vi "Measurement Logic.vi"(8 "error in":errorcluster, 9 "measurement configuration":T2 {"Baudrate" format="%x"; "FD Baudrate" format="%x"}, 10 "measure call context in":refnum<class "Measure Call Context.lvclass">, 11 "Stop OOB Server UE":refnum<user-event>) -> (0 "error out":errorcluster, 1 "measurement results":T1, 2 "measure call context out":refnum<class "Measure Call Context.lvclass">)   [LabVIEW 2025, in "CAN-LIN Raw Bus Capture.lvclass"]
doc: "Contains the core logic for executing the measurement."
uses:
  CAN-LIN Raw Bus Capture.lvclass
  <vilib>/Plug-In SDKs/Measurements/Measure Call Context/Measure Call Context.lvclass
  Measurement Configuration.ctl
  CAN-LIN Raw Bus Capture UI/Toggle.ctl
  Measurement Results.ctl
  <vilib>/xnet/xnet.llb/XNET Read (Frame LIN).vi
  CAN-LIN Raw Bus Capture.lvclass/CAN-LIN Raw Bus Capture.ctl
  <vilib>/xnet/xnet.llb/XNET Read (Frame CAN).vi
  OOB Data Transfer/OOB Data Transfer.lvlib
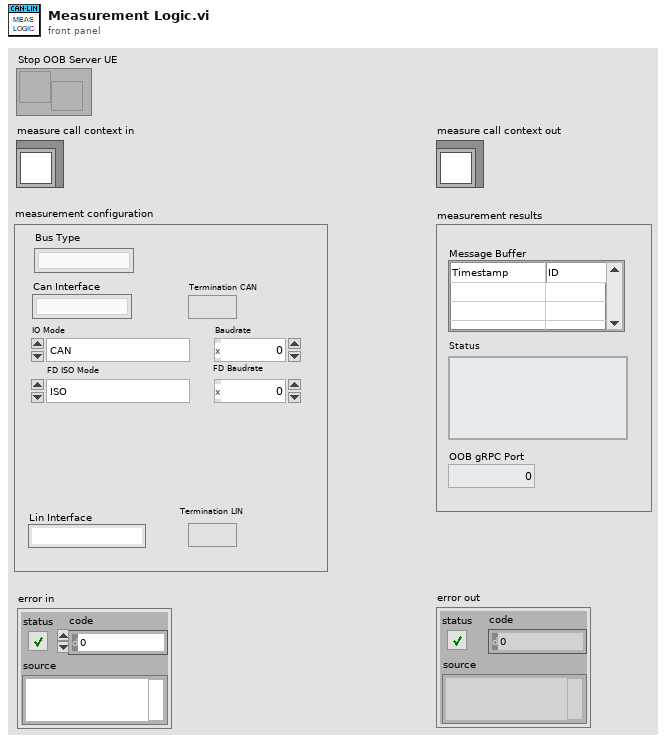
[diagram p1: front panel]
types:
  T1 = typedef "CAN-LIN Raw Bus Capture.lvclass/Measurement Results.ctl" = cluster{"Message Buffer":string[][], "Status":string, "OOB gRPC Port":i32}
  T2 = typedef "CAN-LIN Raw Bus Capture.lvclass/Measurement Configuration.ctl" = cluster{"Termination CAN":T3, "FD Baudrate":u32, "Baudrate":u32, "FD ISO Mode":enum32{"ISO", "Legacy ISO", "Non-ISO"}, "IO Mode":enum32{"CAN", "CAN FD", "CAN FD + BRS"}, "Termination LIN":T3, "Can Interface":string, "Lin Interface":string, "Bus Type":string}
  T3 = typedef "Toggle.ctl" = bool
  T4 = typedef "OOB Data Transfer.lvlib/OOB to Logic Data.ctl" = cluster{"PauseResume":bool, "Export":string}
  T5 = typedef "XNET Frame CAN.ctl" = cluster{"timestamp":timestamp, "payload":u8[], "identifier":u32, "type":T6, "extended?":bool, "echo?":bool}
  T6 = typedef "XNET Frame Type CAN.ctl" = u8
  T7 = typedef "XNET Frame LIN.ctl" = cluster{"timestamp":timestamp, "payload":u8[], "identifier":u32, "type":T8, "event ID":u8, "event slot?":bool, "echo?":bool}
  T8 = typedef "XNET Frame Type LIN.ctl" = u8
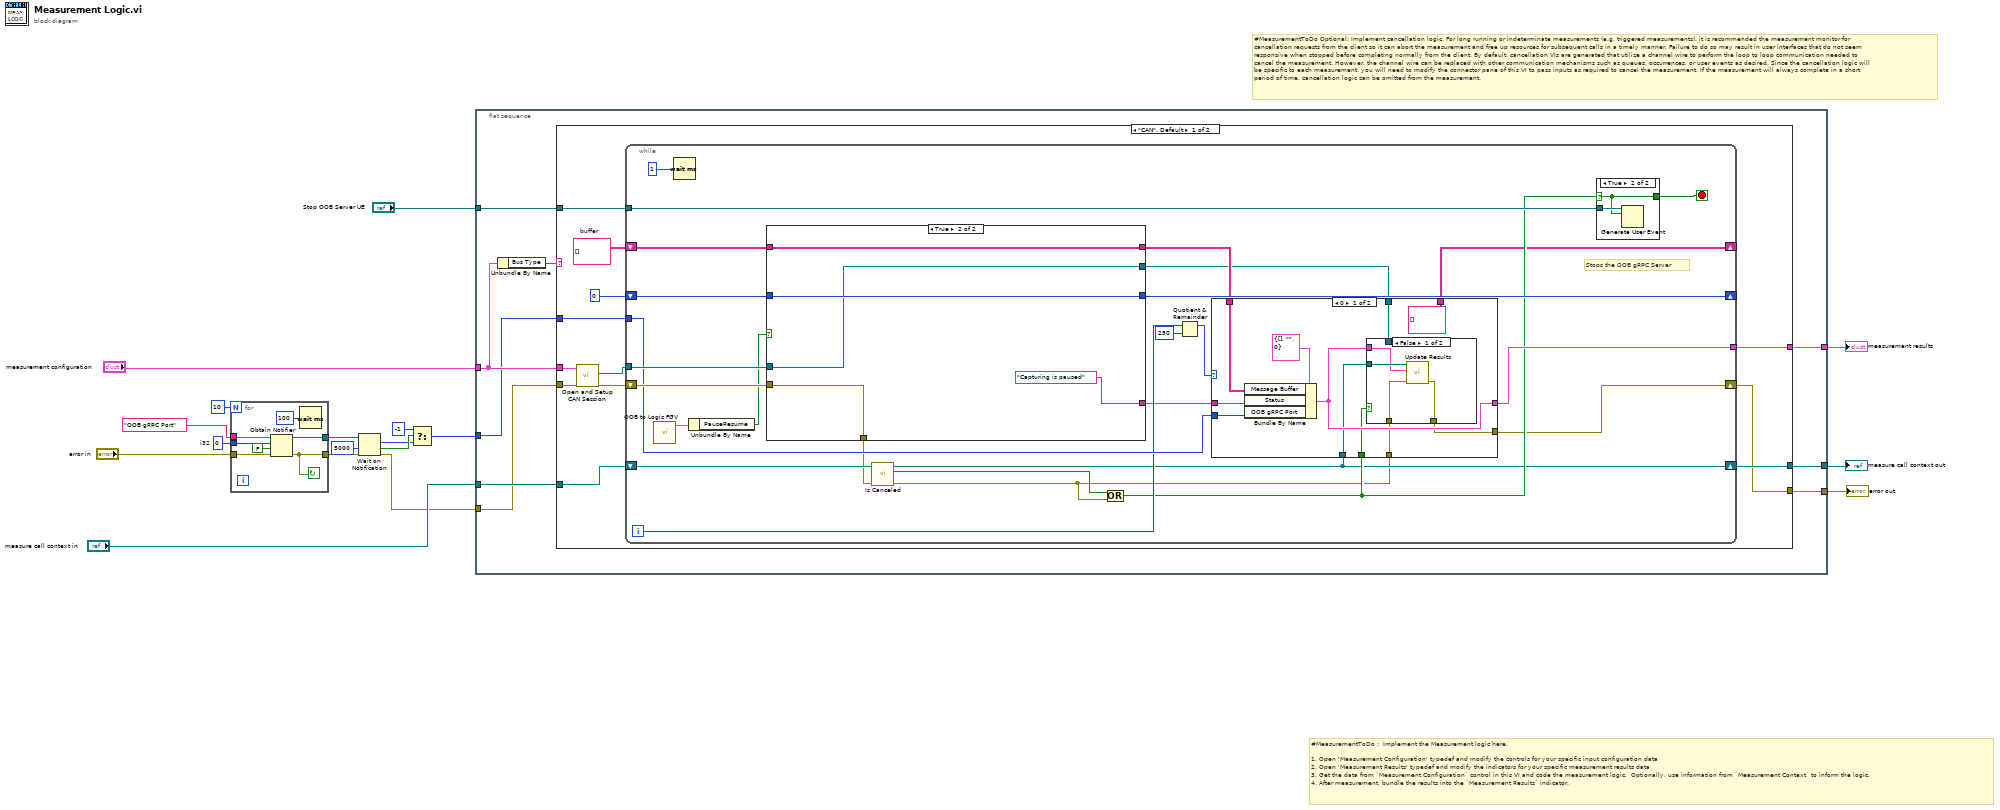
[diagram p0: block diagram]
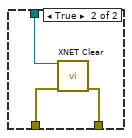
[diagram p2: hidden frame]
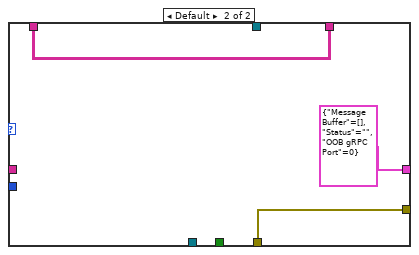
[diagram p3: hidden frame]
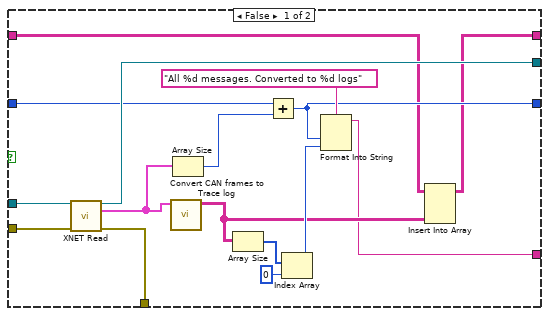
[diagram p4: hidden frame]
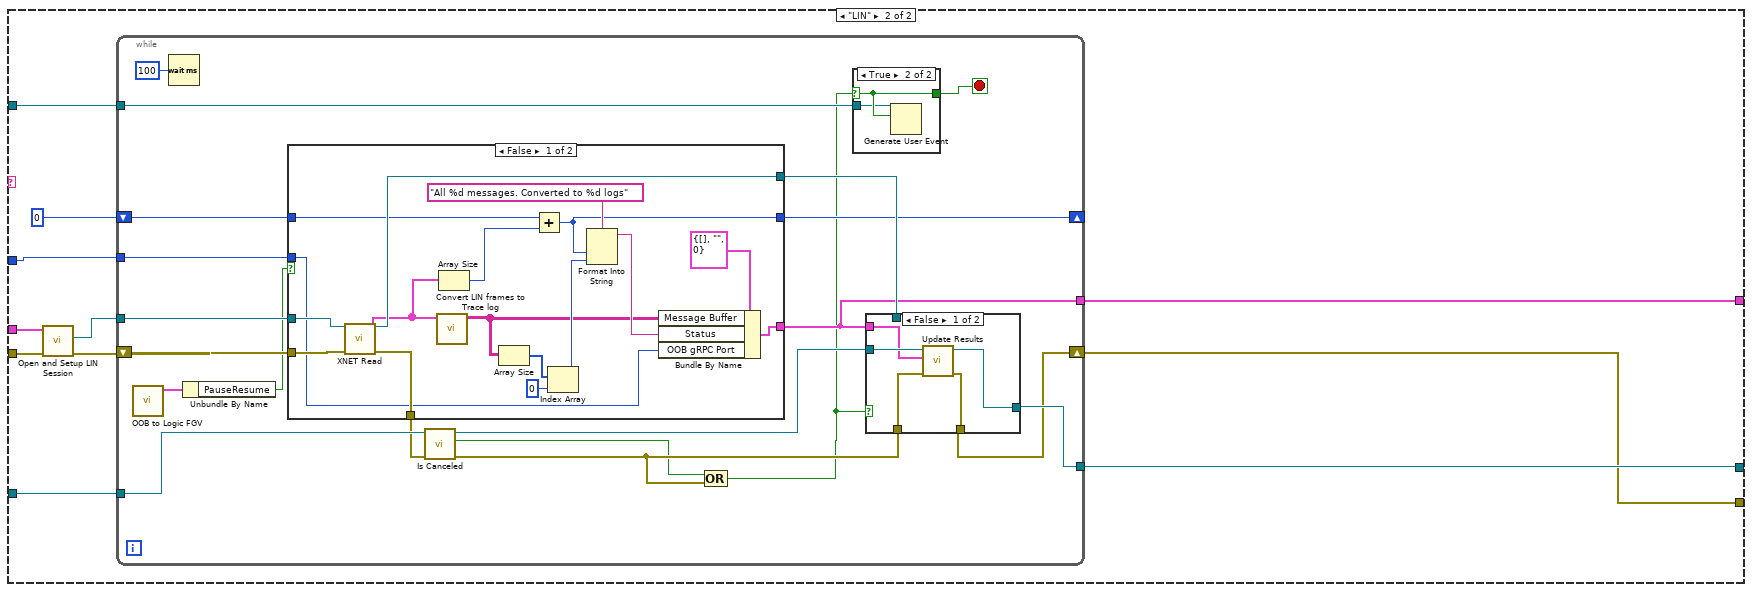
[diagram p6: hidden frame]
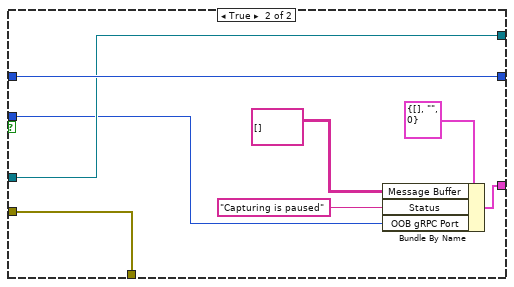
[diagram p8: hidden frame]
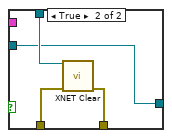
[diagram p9: hidden frame]
diagram:
  w8 = 0  # i32
  # "#MeasurementToDo Optional: Implement cancellation logic. For long running or indeterminate measurements (e.g. triggered measurements), it is recommended the measurement monitor for cancellation requests from the client so it can abort the measurement and free up resources for subsequent calls in a timely manner. Failure to do so may result in user interfaces that do not seem responsive when stopped before completing normally from the client. By default, cancellation VIs are generated that utilize a channel wire to perform the loop to loop communication needed to cancel the measurement. However, the channel wire can be replaced with other communication mechanisms such as queues, occurrences, or user events as desired. Since the cancellation logic will be specific to each measurement, you will need to modify the connector pane of this VI to pass inputs as required to cancel the measurement. If the measurement will always complete in a short period of time, cancellation logic can be omitted from the measurement."
  # "#MeasurementToDo :  Implement the Measurement logic here.\n\n1. Open 'Measurement Configuration' typedef and modify the controls for your specific input configuration data\n2. Open 'Measurement Results' typedef and modify the indicators for your specific measurement results data\n3. Get the data from `Measurement Configuration` control in this VI and code the measurement logic.  Optionally, use information from `Measurement Context` to inform the logic.\n4. After measurement, bundle the results into the `Measurement Results` indicator."
  n1 = for {
    N: 10 -> [_]
    tunnel: [w22] -> w12
    tunnel: [w24] -> w11
    tunnel: "OOB gRPC Port" ("name (unnamed)") -> [w21]
    tunnel: w8 -> [w20]
    tunnel: "error in" -> [w19]
    stop <- w22 continue-if-true
    n2 = Obtain Notifier(name (unnamed)=w21, notification data type=w20, create if not found? (T)=FALSE, error in (no error)=w19) -> (notifier out=w24:refnum<notifier>, error out=w22:errorcluster)  [unwired: 1 out]
    n3 = Wait (ms)(milliseconds to wait=u32 100) -> ()  [unwired: 1 out]
  }
  n4 = Wait on Notification(notifier=w11, timeout in ms (-1)=5000, error in (no error)=w12) -> (notification=w5:i32, timed out?=w6:bool, error out=w2:errorcluster)  [unwired: 1 in, 1 out]
  n5 = Select(t=-1, s=w6, f=w5) -> (s? t:f=w1:i32)
  n6 = flat-sequence {
    tunnel: "measurement configuration" -> [w33]
    tunnel: [w30] -> w17
    tunnel: w2 -> [w31]
    tunnel: "measure call context in" -> [w32]
    tunnel: [w29] -> w15
    tunnel: [w28] -> w14
    tunnel: "Stop OOB Server UE" -> [w27]
    tunnel: w1 -> [w26]
    frame #0 {
      n7 = Unbundle By Name(w33) -> ("Bus Type"=w34:string)
      n8 = case shown="\"CAN\", Default" w34 {
        tunnel: w33 -> [w43 w121]
        tunnel: w32 -> [w42 w124]
        tunnel: w31 -> [w41 w123]
        tunnel: [w40 w125] -> w30
        tunnel: [w39 w127] -> w28
        tunnel: [w38 w126] -> w29
        tunnel: w27 -> [w37 w119]
        tunnel: w26 -> [w36 w118]
        frame "CAN", Default {
          w35 = string[][] []  # buffer
          n9 = call "Open and Setup CAN Session.vi"("error in"=w41, "measurement configuration"=w43) -> ("error out"=w45:errorcluster, "session out"=w46:refnum<k21>)  [unwired: 8 in]
          n10 = while {
            tunnel: [w59] -> w40
            shift-right: [w48] -> w38
            shift-left: w45 -> [w70]
            tunnel: w46 -> [w69]
            shift-right: [w67] -> _
            shift-left: 0 -> [w68]
            tunnel: w37 -> [w66]
            tunnel: w36 -> [w61]
            shift-right: [w51] -> w39
            shift-left: w42 -> [w71]
            shift-right: [w47] -> _
            shift-left: w35 -> [w55]
            i -> [w58]
            stop <- w65 stop-if-true
            # "Stops the OOB gRPC Server"
            n11 = call "OOB to Logic FGV.vi"() -> ("OOB to Logic Data out"=w63:T4)  [unwired: 10 in, 1 out]
            n12 = Wait (ms)(milliseconds to wait=u32 1) -> ()  [unwired: 1 out]
            n13 = Unbundle By Name(w63) -> ("PauseResume"=w62:bool)
            n14 = case shown="True" w62 {
              tunnel: w70 -> [w109 w114]
              tunnel: [w108 w114] -> w60
              tunnel: [w107 w112] -> w49
              tunnel: w69 -> [w106 w112]
              tunnel: w68 -> [w100 w113]
              tunnel: [w98 w113] -> w67
              tunnel: w55 -> [w97 w111]
              tunnel: [w95 w111] -> w54
              tunnel: [w94 "Capturing is paused" ("CAN Bus Info")] -> w53
              frame False {
                n15 = call-poly <vilib>:"XNET Read.vi"("session in"=w106, "error in (no error)"=w109) -> ("session out"=w107:refnum<k21>, "data"=w104:T5[], "error out"=w108:errorcluster)  [unwired: 10 in, 1 out]
                n16 = call "Convert CAN frames to Trace log.vi"("can frames in"=w104) -> ("trace out"=w96:string[][])  [unwired: 10 in]
                n17 = Array Size(array=w104) -> (size(s)=w99:i32)
                n18 = Array Size(array=w96) -> (size(s)=w103:i32[])
                n19 = Add(x=w100, y=w99) -> (x+y=w98:i32)
                n20 = Index Array(array=w103, index=0) -> (element=w101:i32)
                n21 = Format Into String(format string="All %d messages. Converted to %d logs" ("CAN Bus Info"), w98, w101) -> (resulting string=w94:string)  [unwired: 2 in, 1 out]
                n22 = Insert Into Array(array=w97, new element=w96) -> (w95:string[][])  [unwired: 2 in]
              }
              frame True {
              }
            }
            n23 = call <vilib>:"Is Canceled.vi"("error in"=w60, "measure call context in"=w71) -> ("error out"=w50:errorcluster, "is canceled?"=w64:bool, "measure call context out"=w51:refnum<class "Measure Call Context.lvclass">)  [unwired: 7 in]
            n24 = Compound Arithmetic op=OR(w64, w50) -> (w52:bool)
            n25 = Quotient & Remainder(x=w58, y=250) -> (x-y*floor(x/y)=w56:i32)  [unwired: 1 out]
            n26 = case shown="0" w56 {
              tunnel: w61 -> [w82 _]
              tunnel: [w81 T1 {"Message Buffer"=[], "Status"="", "OOB gRPC Port"=0} ("Measurement Results")] -> w59
              tunnel: w54 -> [w80 w91]
              tunnel: w53 -> [w79 _]
              tunnel: w52 -> [w78 _]
              tunnel: w51 -> [w77 _]
              tunnel: w50 -> [w76 w93]
              tunnel: w49 -> [w75 _]
              tunnel: [w74 w93] -> w48
              tunnel: [string[][] [] ("buffer") w91] -> w47
              frame 0 {
                n27 = Bundle By Name(cluster=T1 {"Message Buffer"=[], "Status"="", "OOB gRPC Port"=0} ("Measurement Results"), "Message Buffer"=w80, "Status"=w79, "OOB gRPC Port"=w82) -> (w81:T1)
                n28 = case shown="False" w78 {
                  tunnel: w77 -> [w87 _]
                  tunnel: w76 -> [w86 w90]
                  tunnel: [w85 w89] -> w74
                  tunnel: w75 -> [_ w88]
                  tunnel: w81 -> [w84 _]
                  frame False {
                    n29 = call <vilib>:"Update Results.vi"("error in"=w86, "measurement results"=w84, "measure call context in"=w87) -> ("error out"=w85:errorcluster)  [unwired: 7 in, 1 out]
                  }
                  frame True {
                    n30 = call <vilib>:"XNET Clear.vi"("session in"=w88, "error in (no error)"=w90) -> ("error out"=w89:errorcluster)  [unwired: 13 in]
                  }
                }
              }
              frame Default {
              }
            }
            n31 = case shown="True" w52 {
              selector: w52 -> [w115 w116]
              tunnel: w66 -> [_ w117]
              tunnel: [w115 w116] -> w65
              frame False {
              }
              frame True {
                n32 = Generate User Event(user event=w117, event data cluster=w116) -> ()  [unwired: 2 in, 2 out]
              }
            }
          }
        }
        frame "LIN" {
          n33 = call "Open and Setup LIN Session.vi"("error in"=w123, "measurement configuration"=w121) -> ("error out"=w122:errorcluster, "session out"=w120:refnum<k21>)  [unwired: 8 in]
          n34 = while {
            tunnel: [w142] -> w125
            tunnel: w124 -> [w147]
            tunnel: [w144] -> w127
            shift-right: [w136] -> w126
            shift-left: w122 -> [w146]
            tunnel: w120 -> [w141]
            shift-right: [w139] -> _
            shift-left: 0 -> [w140]
            tunnel: w119 -> [w134]
            tunnel: w118 -> [w130]
            stop <- w135 stop-if-true
            n35 = call "OOB to Logic FGV.vi"() -> ("OOB to Logic Data out"=w138:T4)  [unwired: 10 in, 1 out]
            n36 = Wait (ms)(milliseconds to wait=u32 100) -> ()  [unwired: 1 out]
            n37 = Unbundle By Name(w138) -> ("PauseResume"=w137:bool)
            n38 = case shown="False" w137 {
              tunnel: w146 -> [w167 w171]
              tunnel: [w166 w171] -> w129
              tunnel: [w165 w170] -> w143
              tunnel: [w164 w172] -> w142
              tunnel: w141 -> [w163 w170]
              tunnel: w140 -> [w158 w173]
              tunnel: [w156 w173] -> w139
              tunnel: w130 -> [w152 w169]
              frame False {
                n39 = call-poly <vilib>:"XNET Read.vi"("session in"=w163, "error in (no error)"=w167) -> ("session out"=w165:refnum<k21>, "data"=w154:T7[], "error out"=w166:errorcluster)  [unwired: 10 in, 1 out]
                n40 = call "Convert LIN frames to Trace log.vi"("lin frames in"=w154) -> ("trace out"=w153:string[][])  [unwired: 10 in]
                n41 = Array Size(array=w154) -> (size(s)=w157:i32)
                n42 = Array Size(array=w153) -> (size(s)=w161:i32[])
                n43 = Add(x=w158, y=w157) -> (x+y=w156:i32)
                n44 = Index Array(array=w161, index=0) -> (element=w159:i32)
                n45 = Format Into String(format string="All %d messages. Converted to %d logs" ("CAN Bus Info"), w156, w159) -> (resulting string=w155:string)  [unwired: 2 in, 1 out]
                n46 = Bundle By Name(cluster=T1 {"Message Buffer"=[], "Status"="", "OOB gRPC Port"=0} ("Measurement Results"), "Message Buffer"=w153, "Status"=w155, "OOB gRPC Port"=w152) -> (w164:T1)
              }
              frame True {
                n47 = Bundle By Name(cluster=T1 {"Message Buffer"=[], "Status"="", "OOB gRPC Port"=0} ("Measurement Results"), "Message Buffer"=string[][] [], "Status"="Capturing is paused" ("CAN Bus Info"), "OOB gRPC Port"=w169) -> (w172:T1)
              }
            }
            n48 = call <vilib>:"Is Canceled.vi"("error in"=w129, "measure call context in"=w147) -> ("error out"=w133:errorcluster, "is canceled?"=w132:bool, "measure call context out"=w145:refnum<class "Measure Call Context.lvclass">)  [unwired: 7 in]
            n49 = Compound Arithmetic op=OR(w132, w133) -> (w131:bool)
            n50 = case shown="True" w131 {
              selector: w131 -> [w149 w151]
              tunnel: [w149 w151] -> w135
              tunnel: w134 -> [_ w150]
              frame False {
              }
              frame True {
                n51 = Generate User Event(user event=w150, event data cluster=w151) -> ()  [unwired: 2 in, 2 out]
              }
            }
            n52 = case shown="False" w131 {
              tunnel: w145 -> [w181 w182]
              tunnel: w133 -> [w180 w185]
              tunnel: [w179 w184] -> w136
              tunnel: [w178 w182] -> w144
              tunnel: w143 -> [_ w183]
              tunnel: w142 -> [w177 _]
              frame False {
                n53 = call <vilib>:"Update Results.vi"("error in"=w180, "measurement results"=w177, "measure call context in"=w181) -> ("error out"=w179:errorcluster, "measure call context out"=w178:refnum<class "Measure Call Context.lvclass">)  [unwired: 7 in]
              }
              frame True {
                n54 = call <vilib>:"XNET Clear.vi"("session in"=w183, "error in (no error)"=w185) -> ("error out"=w184:errorcluster)  [unwired: 13 in]
              }
            }
          }
        }
      }
    }
  }
  "error out" <- w15
  "measure call context out" <- w14
  "measurement results" <- w17
